vi "OpenReadSetupFile.vi"(8 "Error In":errorcluster, 11 "Setup File":path) -> (0 "Error Out":errorcluster, 3 "Setup":T1={"Slots"=[], "Memory"=[], "Scan List"="", "Trigger"={"Arm"={"Source"=enum."Hold", "Count"=1, "Infinite?"=FALSE}, "Scan"={"Source"=enum."Hold", "Count"=0, "Infinite?"=FALSE, "Delay (sec)"=0.0, "Interval (sec)"=0.0}, "Channel"={"Source"=enum."Hold", "Count"=0, "Infinite?"=FALSE, "Auto Count?"=FALSE, "Delay (sec)"=0.0, "Interval (sec)"=0.0}}} {"Trigger"."Arm"."Count" min=1 max=99999 step=1})   [LabVIEW 2012]
uses:
  Setup.ctl
  SlotConfiguration.ctl
  BankConfiguration.ctl
  TriggerConfiguration.ctl
  TriggerArmConfiguration.ctl
  driver/Public/Controls/ArmSource.ctl
  TriggerScanConfiguration.ctl
  driver/Public/Controls/ScanSource.ctl
  TriggerChannelConfiguration.ctl
  driver/Public/Controls/TriggerSource.ctl
  <vilib>/xml/Load XML File.vi
  <vilib>/xml/Close Reference(Node).vi
  <vilib>/xml/NI_XML.lvlib
  <resource>/objmgr/DOMUserDefRef.rc
  driver/Keithley-7001.lvlib
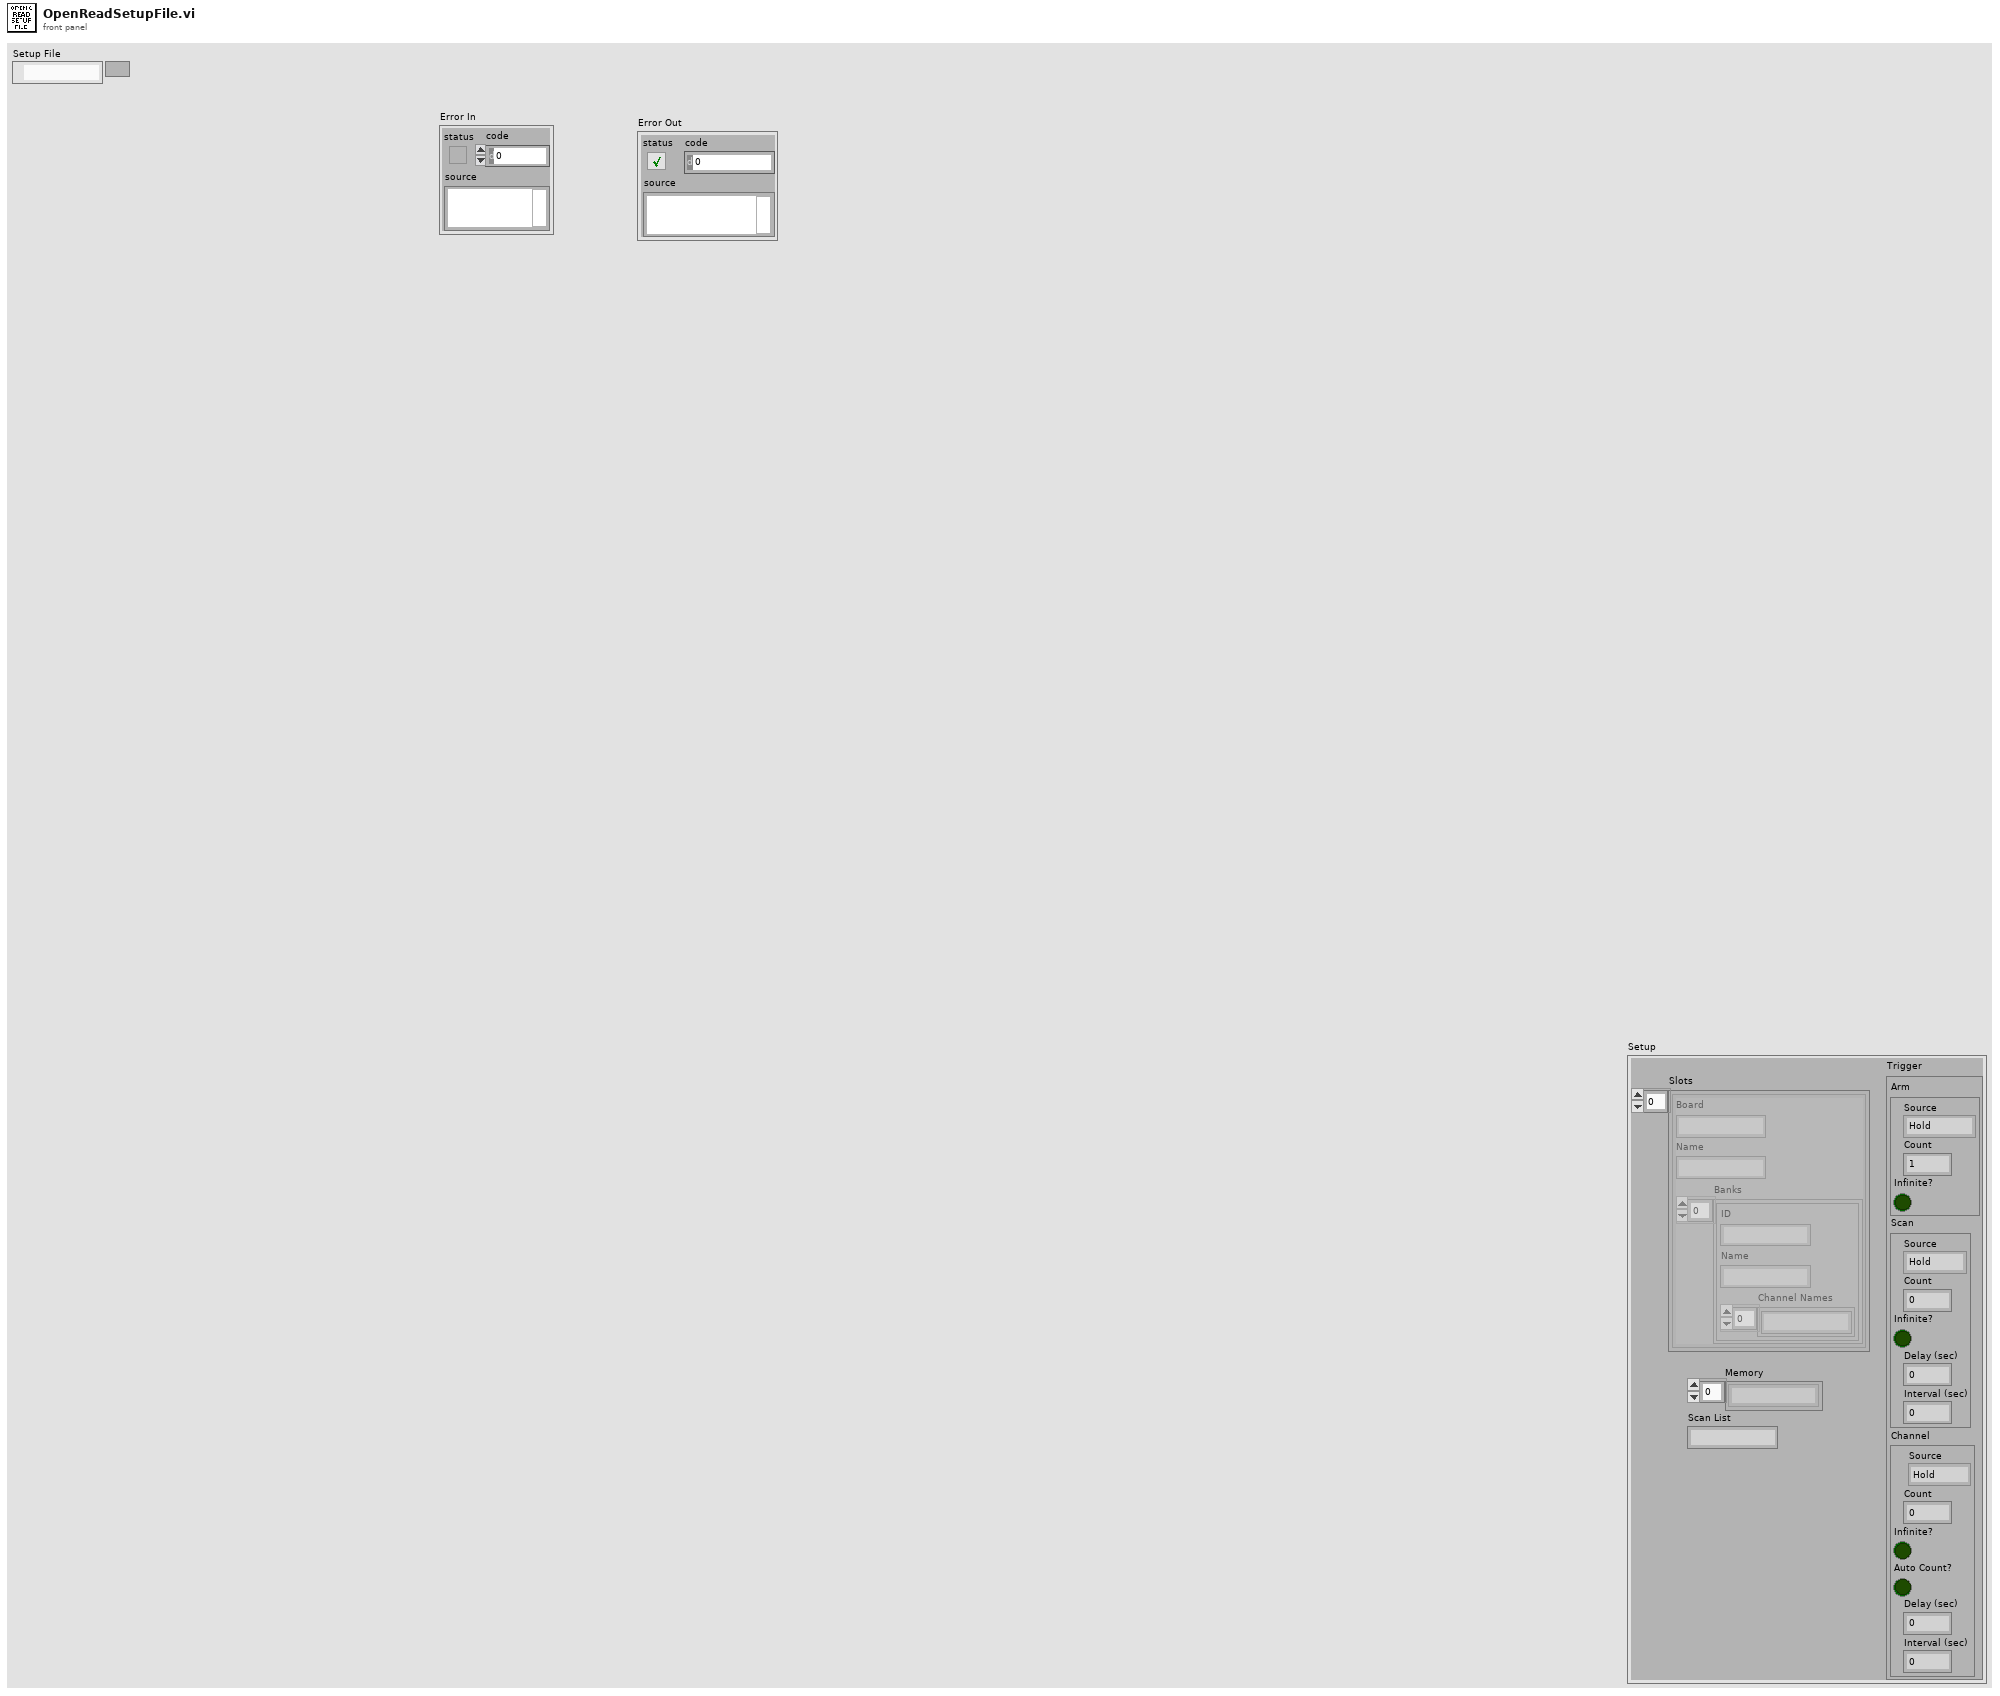
[diagram p1: front panel]
types:
  T1 = typedef "Setup.ctl" = cluster{"Slots":T2[], "Memory":string[], "Scan List":string, "Trigger":T4}
  T2 = typedef "SlotConfiguration.ctl" = cluster{"Board":string, "Name":string, "Banks":T3[]}
  T3 = typedef "BankConfiguration.ctl" = cluster{"ID":string, "Name":string, "Channel Names":string[]}
  T4 = typedef "TriggerConfiguration.ctl" = cluster{"Arm":T5, "Scan":T7, "Channel":T9}
  T5 = typedef "TriggerArmConfiguration.ctl" = cluster{"Source":T6, "Count":u32, "Infinite?":bool}
  T6 = typedef "Keithley-7001.lvlib/ArmSource.ctl" = enum16{"Hold", "Immediate", "Manual", "Bus", "TLink", "External"}
  T7 = typedef "TriggerScanConfiguration.ctl" = cluster{"Source":T8, "Count":u32, "Infinite?":bool, "Delay (sec)":dbl, "Interval (sec)":dbl}
  T8 = typedef "Keithley-7001.lvlib/ScanSource.ctl" = enum16{"Hold", "Immediate", "Timer", "Manual", "Bus", "TLink", "External"}
  T9 = typedef "TriggerChannelConfiguration.ctl" = cluster{"Source":T10, "Count":u32, "Infinite?":bool, "Auto Count?":bool, "Delay (sec)":dbl, "Interval (sec)":dbl}
  T10 = typedef "Keithley-7001.lvlib/TriggerSource.ctl" = enum16{"Hold", "Immediate", "Manual", "Bus", "TLink", "External", "Timer"}
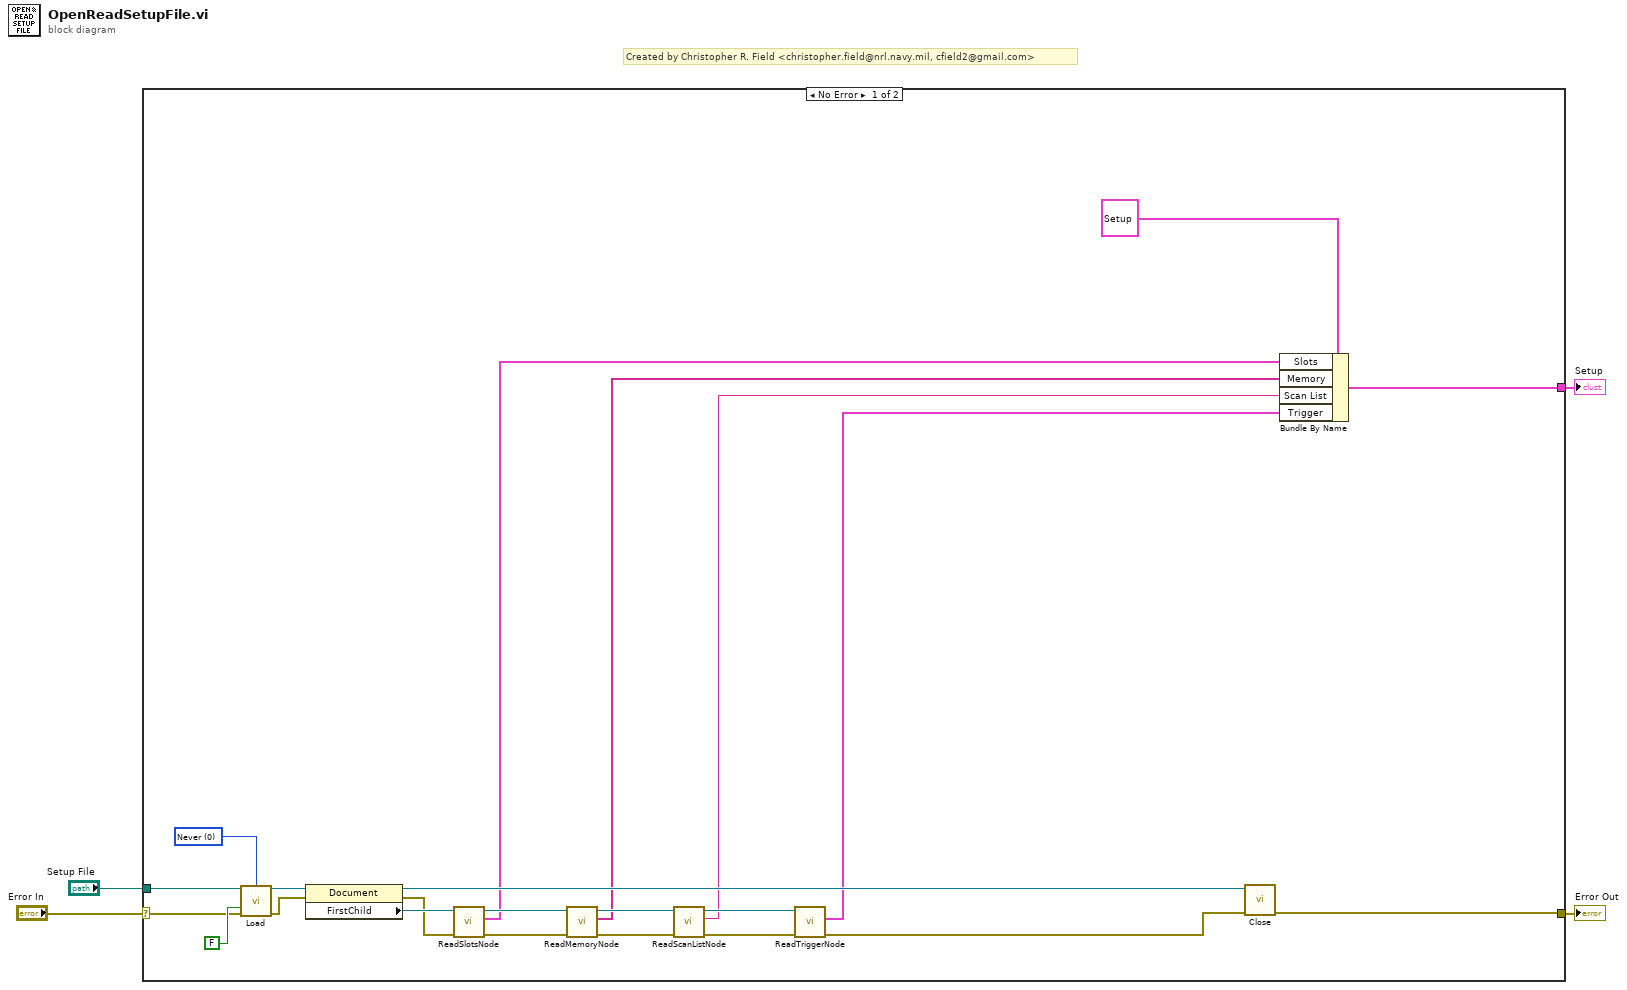
[diagram p0: block diagram]
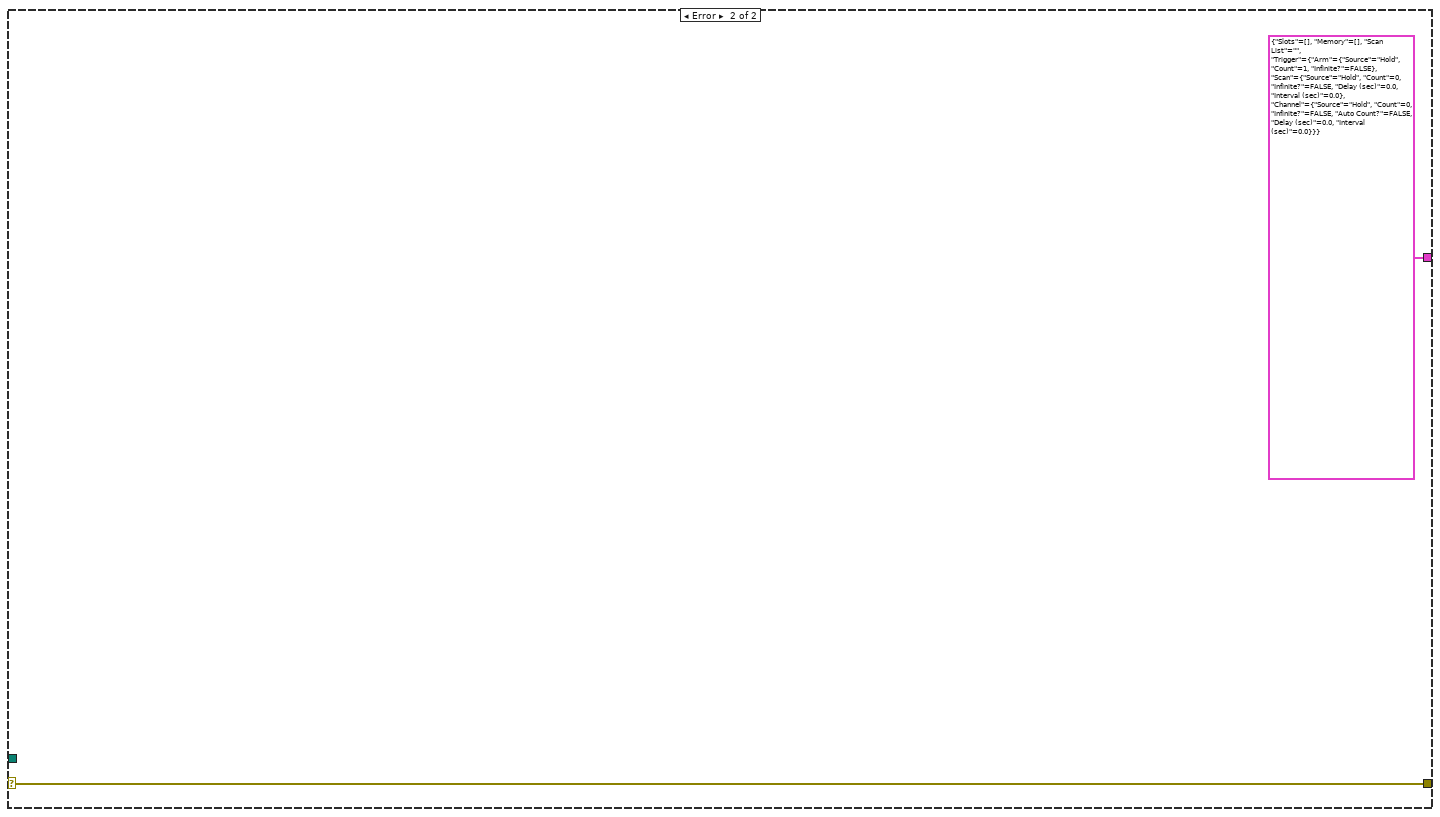
[diagram p2: hidden frame]
diagram:
  # "Created by Christopher R. Field <christopher.field@nrl.navy.mil, cfield2@gmail.com>"
  n1 = case shown="No Error" "Error In" {
    selector: "Error In" -> [w22 w29]
    tunnel: "Setup File" -> [w23 _]
    tunnel: [w20 w29] -> w2
    tunnel: [w5 T1 {"Slots"=[], "Memory"=[], "Scan List"="", "Trigger"={"Arm"={"Source"=enum."Hold", "Count"=1, "Infinite?"=FALSE}, "Scan"={"Source"=enum."Hold", "Count"=0, "Infinite?"=FALSE, "Delay (sec)"=0.0, "Interval (sec)"=0.0}, "Channel"={"Source"=enum."Hold", "Count"=0, "Infinite?"=FALSE, "Auto Count?"=FALSE, "Delay (sec)"=0.0, "Interval (sec)"=0.0}}} ("Setup")] -> w1
    frame No Error {
      w27 = 0 items=["Never", "Always", "Auto"] ("validate on load (Auto)")
      n2 = call-poly <vilib>:"Load.vi"("path to XML document"=w23, "validate on load (Auto)"=w27, "load external DTD (True)"=FALSE, "error in (no error)"=w22) -> ("DOM document out"=w25:refnum<k20>, "error out"=w24:errorcluster)  [unwired: 9 in, 1 out]
      n3 = property class="Document"(reference=w25, error in=w24) -> (reference out=w21:refnum<k20>, error out=w16:errorcluster, "FirstChild"=w19:refnum<k20>)
      n4 = call "ReadSlotsNode.vi"("Error In"=w16, "Multiplexer Node In"=w19) -> ("Error Out"=w17:errorcluster, "Slots"=w9:T2[], "Multiplexer Node Out"=w18:refnum<k20>)  [unwired: 7 in]
      n5 = call "ReadMemoryNode.vi"("Error In"=w17, "Multiplexer Node In"=w18) -> ("Error Out"=w14:errorcluster, "Memory"=w8:string[], "Multiplexer Node Out"=w15:refnum<k20>)  [unwired: 7 in]
      n6 = call "ReadScanListNode.vi"("Error In"=w14, "Multiplexer Node In"=w15) -> ("Error Out"=w12:errorcluster, "Scan List"=w7:string, "Multiplexer Node Out"=w13:refnum<k20>)  [unwired: 7 in]
      n7 = call "ReadTriggerNode.vi"("Error In"=w12, "Multiplexer Node In"=w13) -> ("Error Out"=w11:errorcluster, "Trigger Configuration"=w6:T4)  [unwired: 7 in, 1 out]
      n8 = call-poly <vilib>:"Close.vi"("error in (no error)"=w11, "node"=w21) -> ("error out"=w20:errorcluster)  [unwired: 7 in]
      n9 = Bundle By Name(cluster=T1 {"Slots"=[], "Memory"=[], "Scan List"="", "Trigger"={"Arm"={"Source"=enum."Hold", "Count"=1, "Infinite?"=FALSE}, "Scan"={"Source"=enum."Hold", "Count"=0, "Infinite?"=FALSE, "Delay (sec)"=0.0, "Interval (sec)"=0.0}, "Channel"={"Source"=enum."Hold", "Count"=0, "Infinite?"=FALSE, "Auto Count?"=FALSE, "Delay (sec)"=0.0, "Interval (sec)"=0.0}}} ("Setup"), "Slots"=w9, "Memory"=w8, "Scan List"=w7, "Trigger"=w6) -> (w5:T1)
    }
    frame Error {
    }
  }
  "Error Out" <- w2
  "Setup" <- w1
